vi "Untitled 4.vi"() -> ()   [LabVIEW 2019]
uses:
  <vilib>/myRIO/Instrument Drivers/Onboard IO/PWM/typedefs/PWM Reference.ctl
  <vilib>/myRIO/Common/Instrument Driver Framework/Utilities/typedefs/myRIO Generic Hardware Reference.ctl
  <vilib>/myRIO/Common/Instrument Driver Framework/Utilities/typedefs/Hardware Version Enum.ctl
  <vilib>/myRIO/Common/Instrument Driver Framework/Utilities/typedefs/myRIO v1.0 Reference.ctl
  <vilib>/myRIO/Common/Instrument Driver Framework/Utilities/typedefs/Generic FPGA Reference.ctl
  <vilib>/myRIO/Common/Instrument Driver Framework/myRIO v1.0/PWM/typedefs/PWM Channels Enum.ctl
  <vilib>/myRIO/Instrument Drivers/Onboard IO/PWM/typedefs/PWM Configuration.ctl
  <vilib>/userDefined/High Color/nirio_resource_hc.ctl
  <vilib>/myRIO/Common/Instrument Driver Framework/Utilities/vis/Is FPGA Ref Available.vi
  <vilib>/myRIO/Common/Instrument Driver Framework/myRIO v1.0/PWM/vis/myRIO v1.1 Open PWM.vi
  <vilib>/myRIO/Instrument Drivers/Onboard IO/PWM/vis/Set Duty Cycle and Frequency.vi
  <vilib>/myRIO/Common/Instrument Driver Framework/Utilities/vis/Validate Channels.vi
  <vilib>/myRIO/Common/Instrument Driver Framework/myRIO v1.0/PWM/vis/myRIO v1.0 Reserve PWM.vi
  <vilib>/myRIO/Common/Instrument Driver Framework/myRIO v1.0/PWM/vis/myRIO v1.0 Build MUX Configuration PWM.vi
  <vilib>/myRIO/Common/Instrument Driver Framework/myRIO v1.0/Resource Manager/vis/myRIO v1.0 Reserve Channel List.vi
  <vilib>/myRIO/Common/Instrument Driver Framework/myRIO v1.0/Resource Manager/vis/myRIO v1.0 Create Configuration List.vi
  <vilib>/myRIO/Common/Instrument Driver Framework/myRIO v1.0/Resource Manager/vis/myRIO v1.0 Reserve Channel.vi
  <vilib>/myRIO/Common/Instrument Driver Framework/myRIO v1.0/Resource Manager/vis/myRIO v1.0 Unreserve Channel.vi
  <vilib>/myRIO/Common/Instrument Driver Framework/myRIO v1.0/Resource Manager/vis/myRIO v1.0 Build Mutex Name.vi
  <vilib>/robotics/Kinematics/Generate Joint Trajectory (Int).vi
  <vilib>/Utility/VariantDataType/GetNumericInfo.vi
  <vilib>/Utility/error.llb/Error Cluster From Error Code.vi
  <vilib>/myRIO/Common/Instrument Driver Framework/myRIO v1.0/myRIO v1.1 Open.vi
  <vilib>/myRIO/Common/Instrument Driver Framework/Utilities/vis/IO Manager.vi
  <vilib>/myRIO/Common/Instrument Driver Framework/Utilities/vis/Configuration Manager.vi
  <vilib>/myRIO/Common/Instrument Driver Framework/myRIO v1.0/Resource Manager/vis/myRIO v1.0 Configure IO.vi
  <vilib>/myRIO/Common/Instrument Driver Framework/myRIO v1.0/myRIO v1.0 Close.vi
  <vilib>/myRIO/Common/Instrument Driver Framework/myRIO v1.0/PWM/vis/myRIO v1.0 Write PWM.vi
  <vilib>/myRIO/Express VI/Onboard IO/PWM/PWM Express VI.xnode
  <vilib>/myRIO/Instrument Drivers/Onboard IO/PWM/vis/myRIO PWM Open.xnode
  <vilib>/robotics/Kinematics/NI_Kinematics.lvlib
  <vilib>/myRIO/Instrument Drivers/Onboard IO/PWM/PWM.lvlib
panel:
  in  "start joint positions":dbl[](array[numeric])
  in  "end joint positions":dbl[](array[numeric])
  in  "Slide 6":dbl(slide) scale=0.0..180.0
  in  "Slide 5":dbl(slide) scale=0.0..180.0
  in  "Slide 4":dbl(slide) scale=0.0..180.0
  in  "Slide 3":dbl(slide) scale=0.0..180.0
  in  "Slide 2":dbl(slide) scale=0.0..180.0
  in  "stop":bool
  in  "Slide":dbl(slide) scale=0.0..180.0
  in  "intermediate points":i32
  out "subarray":dbl[](array[numeric])
  out "subarray 2":dbl[](array[numeric])
  in  "array":dbl[](array[numeric])
  out "element":dbl
  out "Waveform Graph":dbl[](graph)
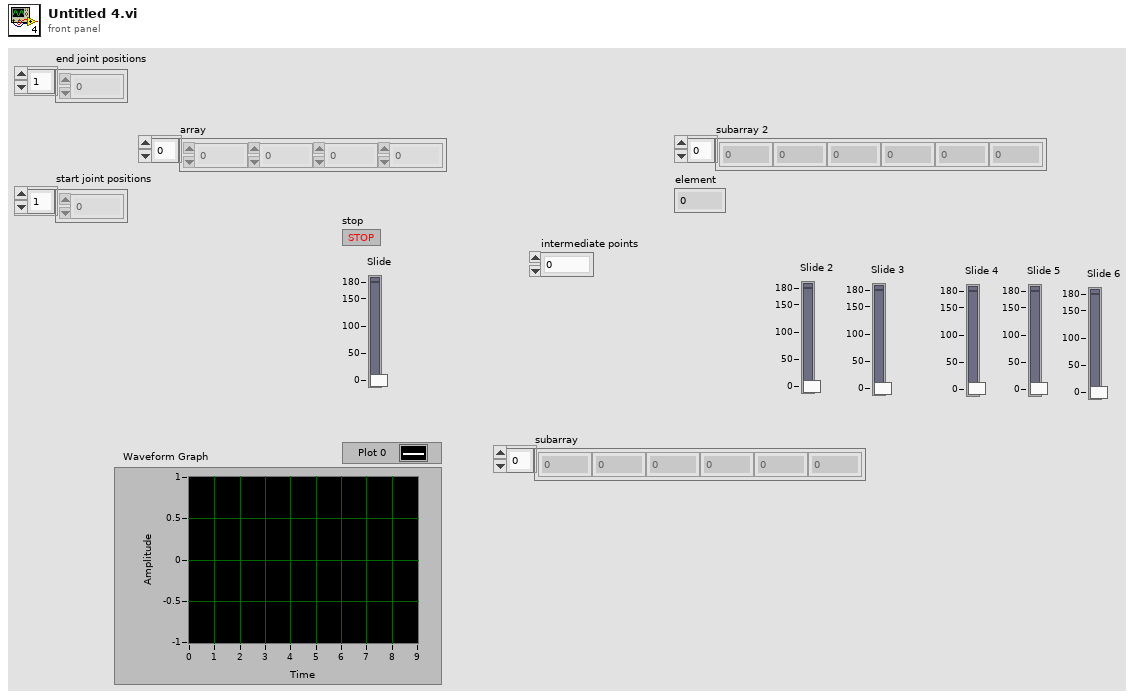
[diagram p1: front panel]
types:
  T1 = typedef "PWM.lvlib/PWM Reference.ctl" = cluster{"myRIO Reference":T2, "PWM Channels Enum":T6, "PWM Configuration":T7}
  T2 = typedef "myRIO Generic Hardware Reference.ctl" = cluster{"myRIO Model":T3, "myRIO Hardware Reference":T4}
  T3 = typedef "Hardware Version Enum.ctl" = enum16{"Unknown", "myRIO-1900", "myRIO-1950", "roboRIO", "NI ELVIS RIO CM", "ELVIS III"}
  T4 = typedef "myRIO v1.0 Reference.ctl" = cluster{"Generic FPGA Reference":T5, "Allow multiple opens":bool}
  T5 = typedef "Generic FPGA Reference.ctl" = refnum<k20>
  T6 = typedef "PWM Channels Enum.ctl" = enum16{"Not Connected", "C/PWM0", "C/PWM1", "A/PWM0", "A/PWM1", "A/PWM2", "A/PWM3", "A/PWM4", "A/PWM5", "A/PWM6", "A/PWM7", "A/PWM8", "A/PWM9", "A/PWM10", "A/PWM11", "A/PWM12", "A/PWM13", "A/PWM14", "A/PWM15", "A/PWM16", "A/PWM17", "A/PWM18", "A/PWM19", "B/PWM0", "B/PWM1", "B/PWM2", "B/PWM3", "B/PWM4", "B/PWM5", "B/PWM6", "B/PWM7", "B/PWM8", "B/PWM9", "B/PWM10", "B/PWM11", "B/PWM12", "B/PWM13", "B/PWM14", "B/PWM15", "B/PWM16", "B/PWM17", "B/PWM18", "B/PWM19", "PWM/PWM0", "PWM/PWM1", "PWM/PWM2", "PWM/PWM3", "PWM/PWM4", "PWM/PWM5", "PWM/PWM6", "PWM/PWM7", "PWM/PWM8", "PWM/PWM9"}
  T7 = typedef "PWM.lvlib/PWM Configuration.ctl" = cluster{"Frequency":dbl, "Duty Cycle":dbl}
  T8 = typedef "nirio_resource_hc.ctl" = tag
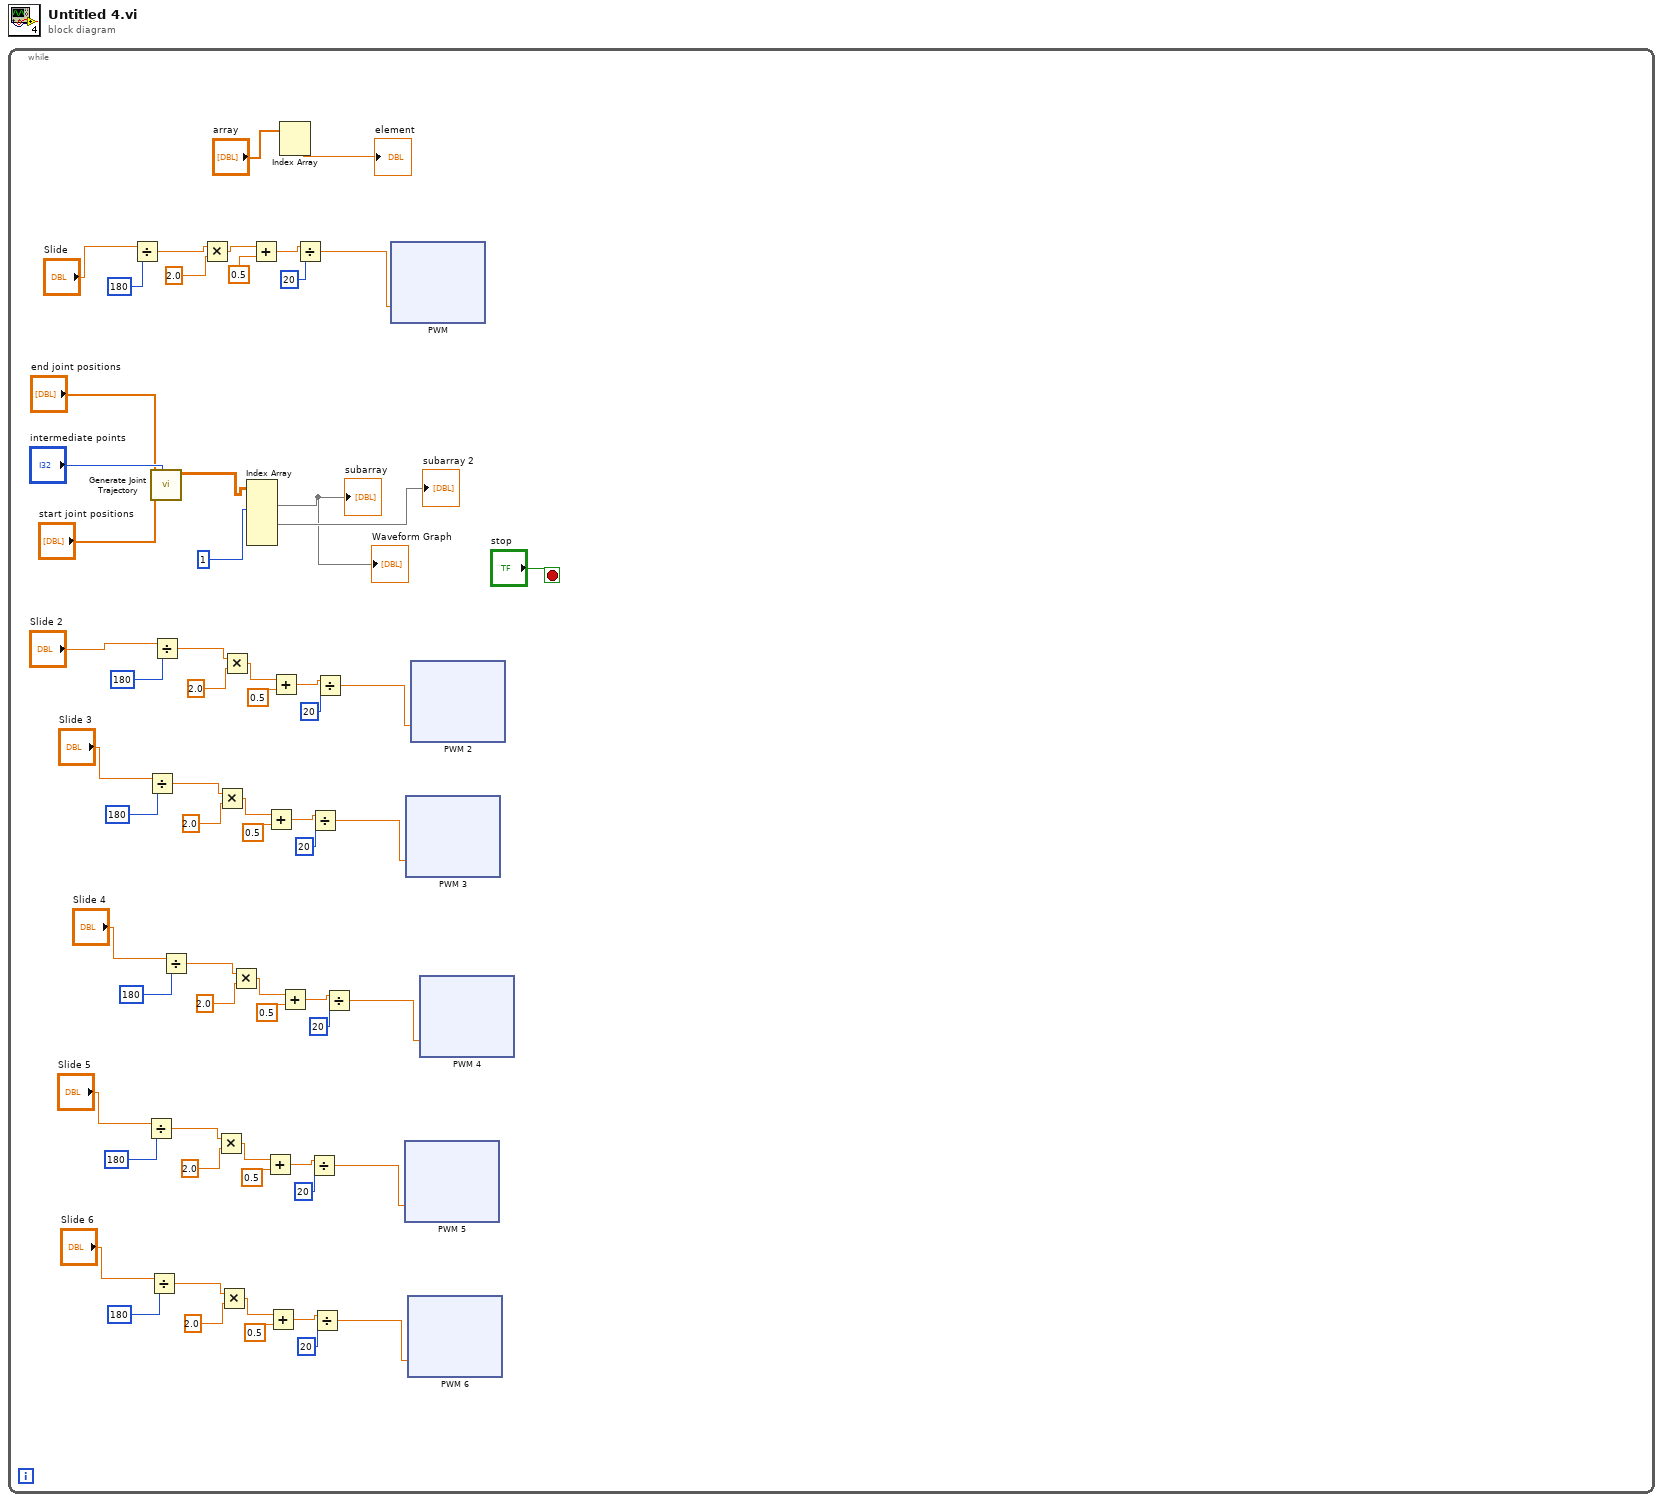
[diagram p0: block diagram]
diagram:
  n1 = while {
    stop <- "stop" stop-if-true
    n2 = Divide(x="Slide", y=180) -> (x/y=w60:dbl)
    n3 = Divide(x="Slide 5", y=180) -> (x/y=w18:dbl)
    n4 = Divide(x="Slide 3", y=180) -> (x/y=w36:dbl)
    n5 = Divide(x="Slide 6", y=180) -> (x/y=w9:dbl)
    n6 = call-poly <vilib>:"Generate Joint Trajectory.vi"("intermediate points"="intermediate points", "end joint positions"="end joint positions", "start joint positions"="start joint positions") -> ("joint position trajectory"=w49:dbl[][])  [unwired: 5 in, 3 out]
    n7 = Divide(x="Slide 2", y=180) -> (x/y=w45:dbl)
    n8 = Divide(x="Slide 4", y=180) -> (x/y=w27:dbl)
    n9 = Multiply(x=w60, y=2.0) -> (x*y=w62:dbl)
    n10 = Multiply(x=w18, y=2.0) -> (x*y=w20:dbl)
    n11 = Multiply(x=w36, y=2.0) -> (x*y=w38:dbl)
    n12 = Multiply(x=w9, y=2.0) -> (x*y=w11:dbl)
    n13 = Multiply(x=w45, y=2.0) -> (x*y=w47:dbl)
    n14 = Multiply(x=w27, y=2.0) -> (x*y=w29:dbl)
    n15 = Index Array "Index Array"(array=w49, index (col) #1=1) -> (element #1=→"subarray" →"Waveform Graph":dbl[], element #2=→"subarray 2":dbl[])  [unwired: 5 in, 1 out]
    n16 = Add(x=w62, y=0.5) -> (x+y=w57:dbl)
    n17 = Add(x=w20, y=0.5) -> (x+y=w15:dbl)
    n18 = Add(x=w38, y=0.5) -> (x+y=w33:dbl)
    n19 = Add(x=w11, y=0.5) -> (x+y=w6:dbl)
    n20 = Add(x=w47, y=0.5) -> (x+y=w42:dbl)
    n21 = Index Array(array="array") -> (element #1=→"element":dbl)  [unwired: 2 in, 1 out]
    n22 = Add(x=w29, y=0.5) -> (x+y=w24:dbl)
    n23 = Divide(x=w57, y=20) -> (x/y=w55:dbl)
    n24 = Divide(x=w15, y=20) -> (x/y=w13:dbl)
    n25 = Divide(x=w33, y=20) -> (x/y=w31:dbl)
    n26 = Divide(x=w6, y=20) -> (x/y=w4:dbl)
    n27 = Divide(x=w42, y=20) -> (x/y=w40:dbl)
    n28 = Divide(x=w24, y=20) -> (x/y=w22:dbl)
    n29 = xnode "PWM"("Duty Cycle"=w55) -> ()  [unwired: 1 in, 1 out]
    n30 = xnode "PWM 5"("Duty Cycle"=w13) -> ()  [unwired: 1 in, 1 out]
    n31 = xnode "PWM 3"("Duty Cycle"=w31) -> ()  [unwired: 1 in, 1 out]
    n32 = xnode "PWM 6"("Duty Cycle"=w4) -> ()  [unwired: 1 in, 1 out]
    n33 = xnode "PWM 2"("Duty Cycle"=w40) -> ()  [unwired: 1 in, 1 out]
    n34 = xnode "PWM 4"("Duty Cycle"=w22) -> ()  [unwired: 1 in, 1 out]
  }
